vi "GE 5565PIORC.PIO.Write (1D Bool).vi"(8 "error in (no error)":errorcluster, 9 "data":bool[](array[boolean]), 10 "offset":u32, 11 "GE 5565PIORC in":refnum<class "GE 5565PIORC.lvclass">) -> (0 "error out":errorcluster, 1 "data out":bool[](array[boolean]), 3 "GE 5565PIORC out":refnum<class "GE 5565PIORC.lvclass">)   [LabVIEW 2016, in "GE 5565PIORC.lvclass"]
doc: "Writes the contents of <B>data</B> to the specified <B>offset</B>. The number of elements transferred will be the number of elements in <B>data</B>."
uses:
  GE 5565PIORC.lvclass
  <vilib>/Instr/_visa.llb/VISA Register Access Address Space.ctl
  GE 5565PIORC.lvclass/GE 5565PIORC.ctl
  GE 5565PIORC.VISA.Move Out.String (U8).vi
  GE 5565PIORC.VISA.Return Handler.vi
  <vilib>/Utility/error.llb/Error Cluster From Error Code.vi
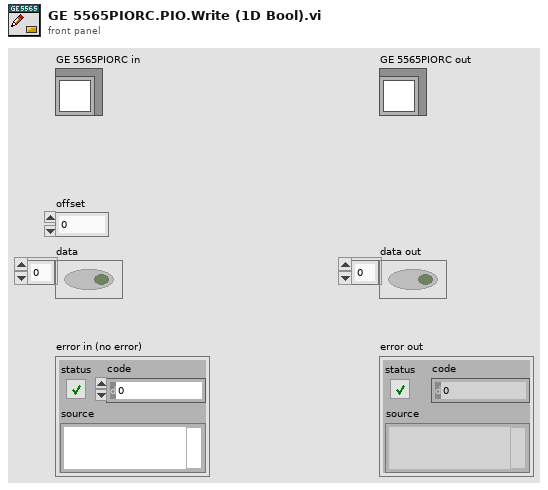
[diagram p1: front panel]
types:
  T1 = typedef "VISA Register Access Address Space.ctl" = u16
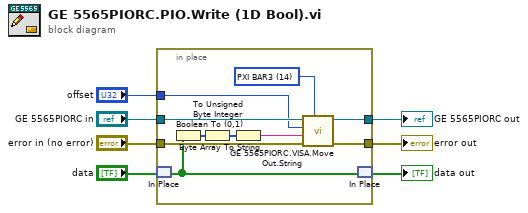
[diagram p0: block diagram]
diagram:
  n1 = in-place {
    in-place-border: "error in (no error)" -> [w12]
    in-place-border: [w15] -> w6
    in-place-border: "GE 5565PIORC in" -> [w16]
    in-place-border: "offset" -> [w14]
    in-place-border: [w13] -> w1
    w17 = T1 14 items=["VXI/VME A16"=1, "VXI/VME A24"=2, "VXI/VME A32"=3, "VXI/VME A64"=4, "PXI Memory Allocations"=9, "PXI Configuration"=10, "PXI BAR0"=11, "PXI BAR1"=12, "PXI BAR2"=13, "PXI BAR3"=14, "PXI BAR4"=15, "PXI BAR5"=16] ("address space")
    n2 = in-place-match #1("data") -> (w9:bool[])
    n3 = Boolean To (0,1)(Boolean=w9) -> (0, 1=w10:i16[])
    n4 = To Unsigned Byte Integer(number=w10) -> (unsigned 8bit integer=w8:u8[])
    n5 = Byte Array To String(unsigned byte array=w8) -> (string=w11:string)
    n6 = call-poly "GE 5565PIORC.VISA.Move Out.String.vi"("address space"=w17, "error in (no error)"=w12, "data in"=w11, "offset"=w14, "GE 5565PIORC in"=w16) -> ("error out"=w15:errorcluster, "GE 5565PIORC out"=w13:refnum<class "GE 5565PIORC.lvclass">)  [unwired: 4 in, 1 out]
    n7 = in-place-match #1(w9) -> (→"data out":bool[])
  }
  "GE 5565PIORC out" <- w1
  "error out" <- w6
